vi "Control_laser_Main.vi"() -> ()   [LabVIEW 2024]
doc: "Use this template to build a simple state machine design pattern. Each state executes code and determines which state to transition to."
uses:
  controls/main_control State.ctl
  controls/main_control Data.ctl
  <vilib>/Utility/error.llb/DialogType.ctl
  <vilib>/DAQmx/create/channels.llb/DAQmx Create Channel (AI-Voltage-Basic).vi
  <vilib>/Utility/error.llb/Error Cluster From Error Code.vi
  <vilib>/ErrorRing/Error Ring.xnode
panel:
  in  "Laser diode control":bool
  out "Sweep Chart":dbl(graph)
  out "Laser Current (mA)":dbl
  out "Data Acq Iterations":i32
  in  "Connect DAQ":bool
  in  "Connect LD Control":bool
  out "Static acquisition Chart":dbl(graph)
  out "Standard deviation":dbl
  out "Mean":dbl
  in  "Mean iterations":i32
  in  "Stop Sweep":bool
  out "Sweep Running":bool
  out "Current Step":dbl format="%#_13g"
  in  "Final value (mA)":dbl format="%#_13g"
  in  "Interval (mA)":dbl format="%#_13g"
  in  "Initial value (mA)":dbl format="%#_13g"
  in  "Init Sweep":bool
  out "Steps":dbl format="%#_13g"
  in  "Data Acquisition":bool
  in  "Exit":bool
  in  "CH. AI Input":tag
  # "SWEEP PARAMETERS"
  # "STATIC ACQUISITION"
  # "LASER"
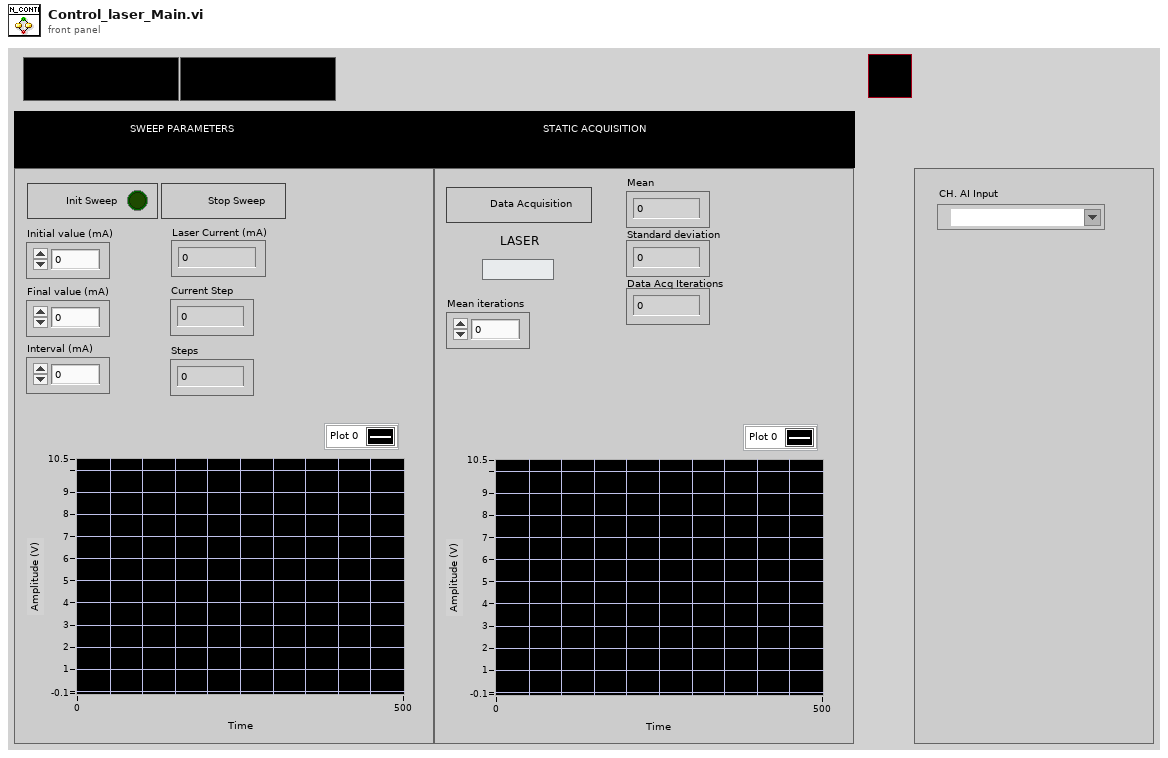
[diagram p1: front panel]
types:
  T1 = cluster{"Steps":refnum<vi>, "Current Step":refnum<vi>, "Final value (mA)":refnum<vi>, "Initial value (mA)":refnum<vi>, "Interval (mA)":refnum<vi>, "Data Acquisition":refnum<vi>, "Init Sweep":refnum<vi>, "Sweep Running":refnum<vi>, "Connect DAQ":refnum<vi>, "Connect LD Control":refnum<vi>}
  T2 = typedef "main_control Data.ctl" = cluster{"Boolean <Replace Me>":bool, "State":string, "Numeric <Replace Me>":dbl}
  T3 = typedef "main_control State.ctl" = enum16{"Initialize", "DAQ Handler", "LD Handler", "Wait for Event", "Data Acquisition", "Freq Sweep (Current)", "Error", "Exit"}
  T4 = typedef "DialogType.ctl" = u16
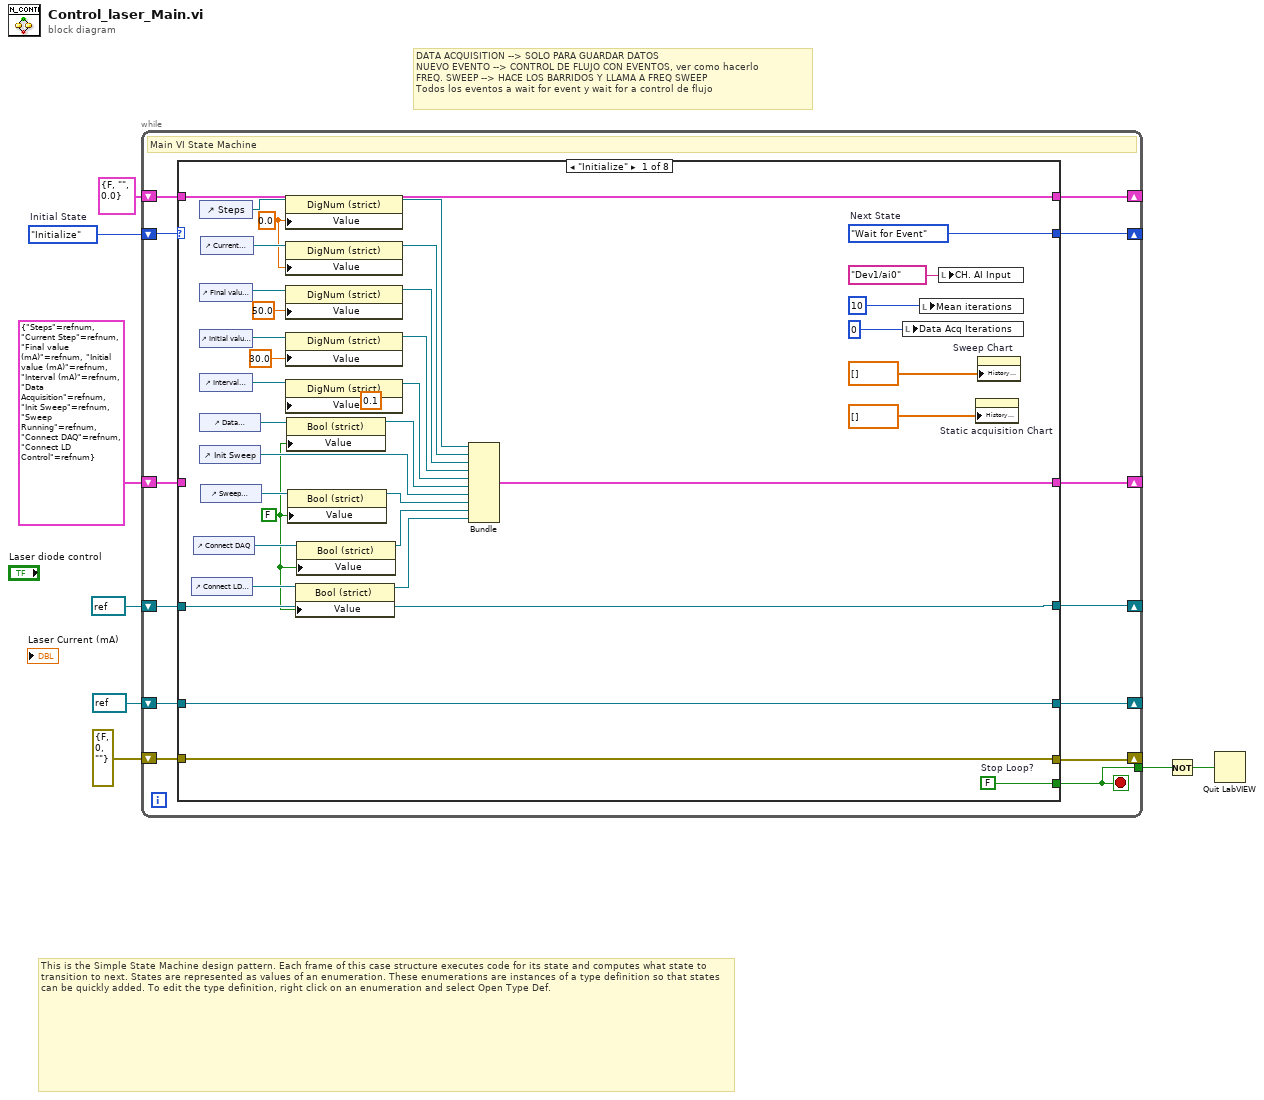
[diagram p0: block diagram]
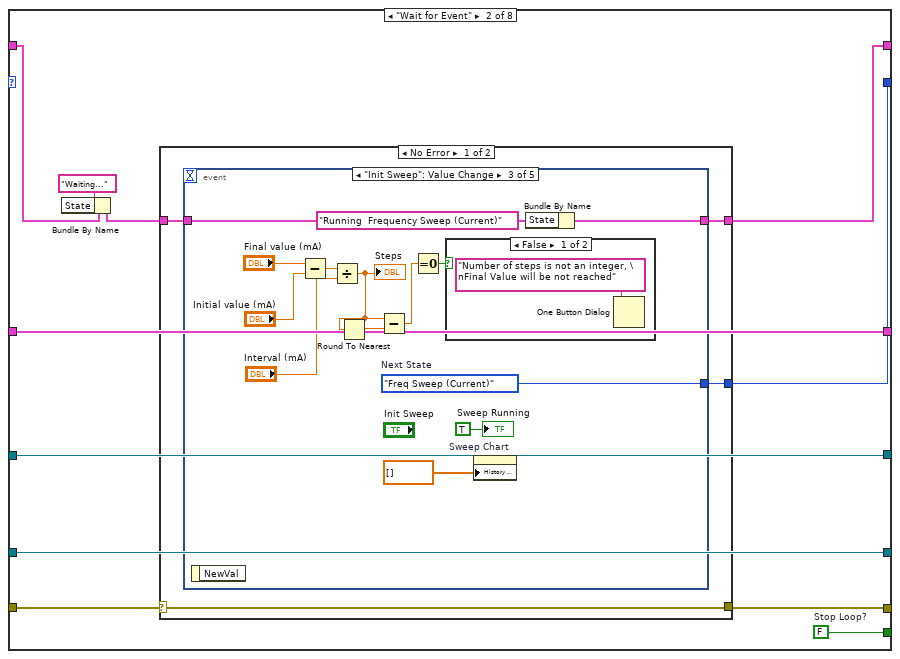
[diagram p2: hidden frame]
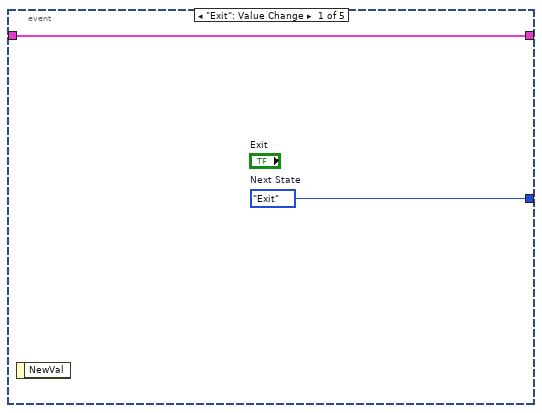
[diagram p3: hidden frame]
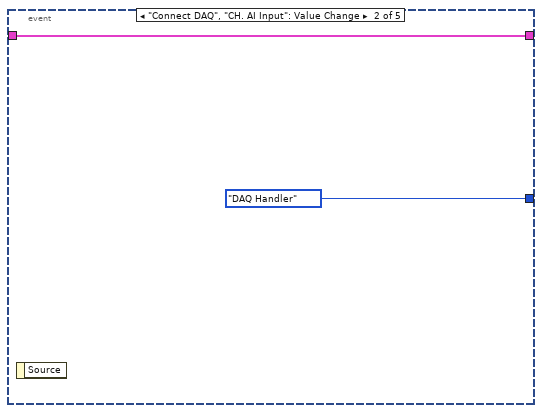
[diagram p4: hidden frame]
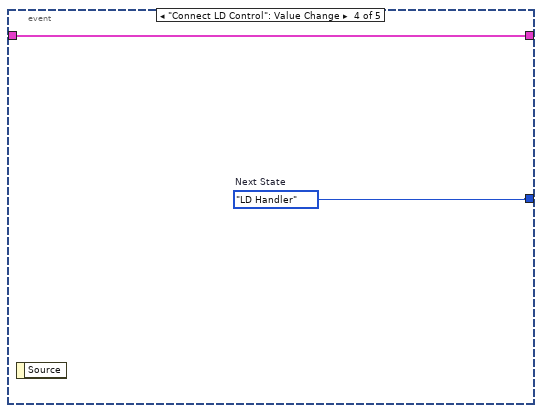
[diagram p6: hidden frame]
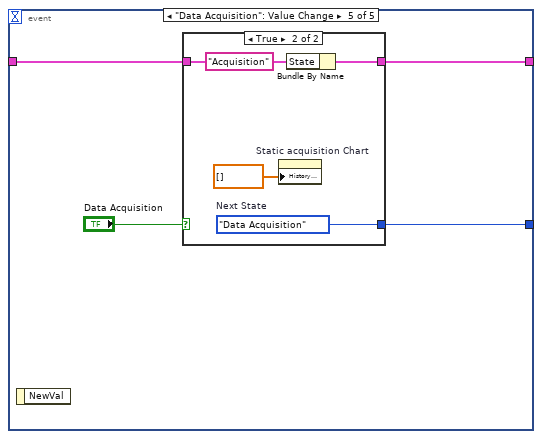
[diagram p7: hidden frame]
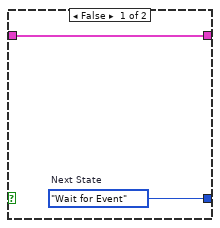
[diagram p8: hidden frame]
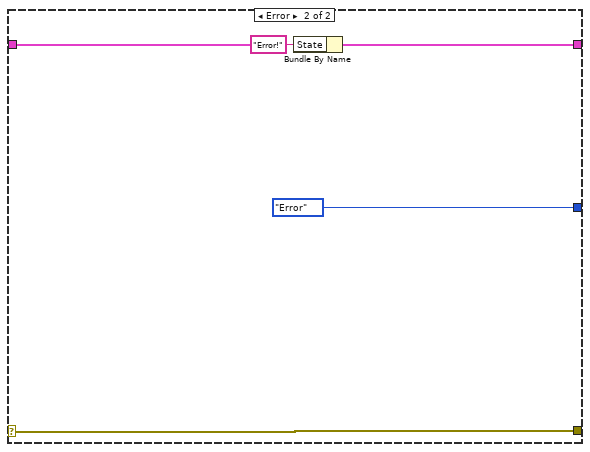
[diagram p9: hidden frame]
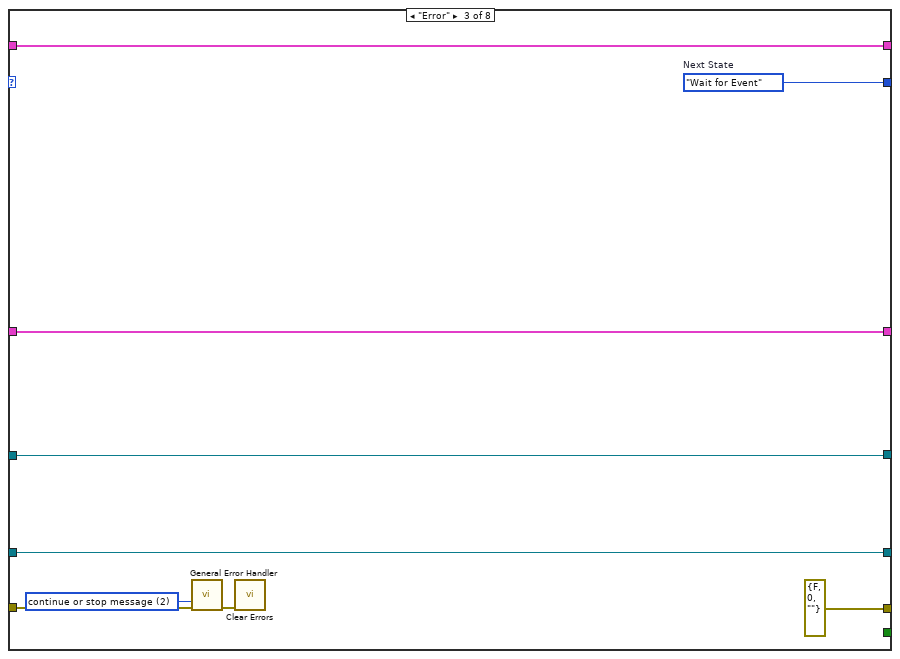
[diagram p10: hidden frame]
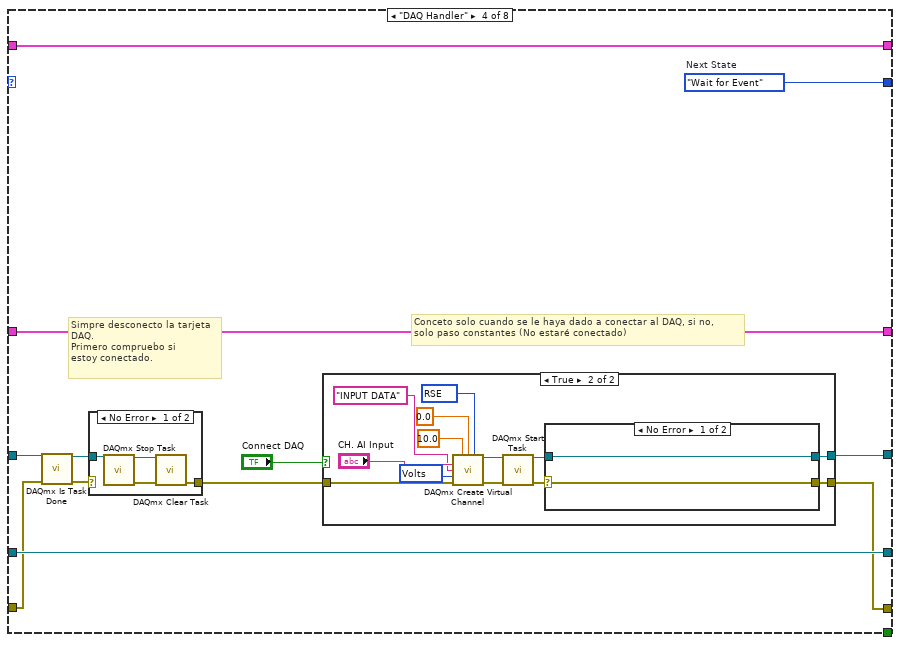
[diagram p11: hidden frame]
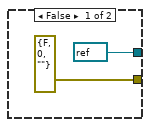
[diagram p12: hidden frame]
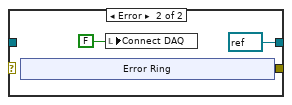
[diagram p13: hidden frame]
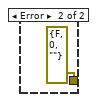
[diagram p14: hidden frame]
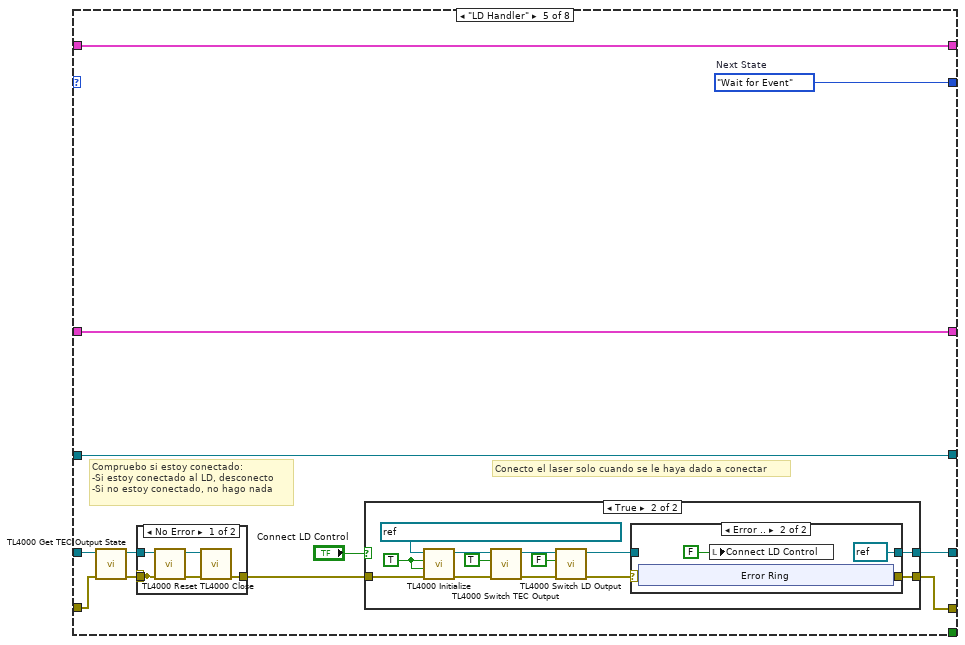
[diagram p15: hidden frame]
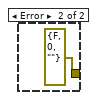
[diagram p16: hidden frame]
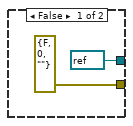
[diagram p17: hidden frame]
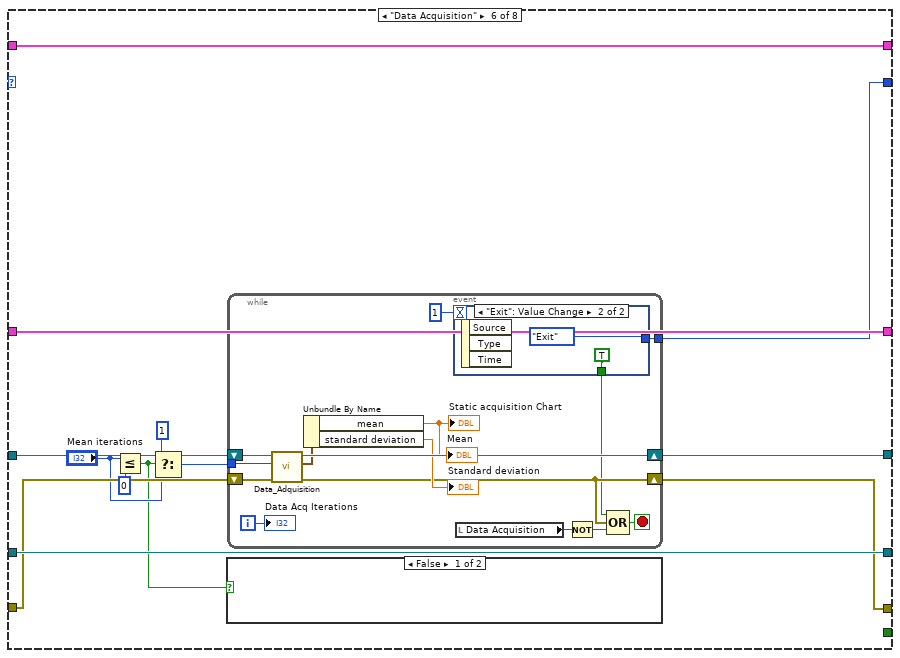
[diagram p19: hidden frame]
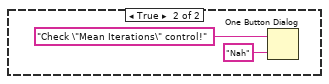
[diagram p20: hidden frame]
diagram:
  w8 = main_control_State."Initialize"  # Initial State
  # "DATA ACQUISITION --> SOLO PARA GUARDAR DATOS\nNUEVO EVENTO --> CONTROL DE FLUJO CON EVENTOS, ver como hacerlo\nFREQ. SWEEP --> HACE LOS BARRIDOS Y LLAMA A FREQ SWEEP\nTodos los eventos a wait for event y wait for a control de flujo"
  # "This is the Simple State Machine design pattern. Each frame of this case structure executes code for its state and computes what state to transition to next. States are represented as values of an enumeration. These enumerations are instances of a type definition so that states can be quickly added. To edit the type definition, right click on an enumeration and select Open Type Def."
  n1 = while {
    shift-right: [w20] -> _
    shift-left: w8 -> [w21]
    shift-right: [w18] -> _
    shift-left: T2 {"Boolean <Replace Me>"=FALSE, "State"="", "Numeric <Replace Me>"=0.0} ("Data") -> [w19]
    shift-right: [w17] -> _
    shift-left: refnum<visa-resource-name> refnum ("instrument handle out") -> [w14]
    shift-right: [w16] -> _
    shift-left: errorcluster {"status"=FALSE, "code"=0, "source"=""} ("error out") -> [w15]
    shift-right: [w12] -> _
    shift-left: T1 {"Steps"=refnum, "Current Step"=refnum, "Final value (mA)"=refnum, "Initial value (mA)"=refnum, "Interval (mA)"=refnum, "Data Acquisition"=refnum, "Init Sweep"=refnum, "Sweep Running"=refnum, "Connect DAQ"=refnum, "Connect LD Control"=refnum} -> [w13]
    shift-right: [w11] -> _
    shift-left: refnum<k21> refnum ("task out") -> [w10]
    tunnel: [w9] -> w3
    stop <- w9 stop-if-true
    # "Main VI State Machine"
    n2 = case shown="\"Initialize\"" w21 {
      tunnel: [w57 w68 w110 w127 w168 w211 w254 w316] -> w20
      tunnel: [w56 w67 _ _ _ _ _ w314] -> w9
      tunnel: w19 -> [w28 w59 w118 w130 w172 w216 w258 w315]
      tunnel: [w28 w66 w118 w130 w172 w216 w259 w315] -> w18
      tunnel: [w37 w65 w113 w128 w171 w214 w246 refnum<visa-resource-name> refnum ("VISA Refnum out")] -> w17
      tunnel: [w36 w61 errorcluster {"status"=FALSE, "code"=0, "source"=""} ("error IO") w120 w170 w209 w244 w312] -> w16
      tunnel: w15 -> [w36 w62 w117 w123 w166 w210 w252 w305]
      tunnel: w14 -> [w37 w65 w113 w128 w167 w214 w250 w308]
      tunnel: [w40 w63 w111 w121 w161 w215 w257 w313] -> w12
      tunnel: w13 -> [_ w63 w111 w121 w161 w215 w257 w313]
      tunnel: [w35 w64 w112 w129 w169 w213 w256 refnum<k21> refnum ("task out")] -> w11
      tunnel: w10 -> [w35 w64 w112 w125 w169 w212 w255 w303]
      frame "Initialize" {
        w24 = FALSE ("Value")
        w47 = 0.0
        w56 = FALSE  # Stop Loop?
        w57 = main_control_State."Wait for Event"  # Next State
        # "Initialize - Initialize the application."
        n3 = control-ref of="Connect LD Control"() -> (w25:refnum<vi>)
        n4 = control-ref of="Connect DAQ"() -> (w34:refnum<vi>)
        n5 = control-ref of="Steps"() -> (w55:refnum<vi>)
        n6 = control-ref of="Final value (mA)"() -> (w54:refnum<vi>)
        n7 = control-ref of="Initial value (mA)"() -> (w53:refnum<vi>)
        n8 = control-ref of="Interval (mA)"() -> (w52:refnum<vi>)
        n9 = control-ref of="Data Acquisition"() -> (w33:refnum<vi>)
        n10 = control-ref of="Init Sweep"() -> (w41:refnum<vi>)
        n11 = control-ref of="Current Step"() -> (w48:refnum<vi>)
        n12 = control-ref of="Sweep Running"() -> (w39:refnum<vi>)
        n13 = property class="DigNum (strict)"(reference=w55, "Value"=w47) -> (reference out=w46:refnum<vi>)  [unwired: 1 in, 1 out]
        n14 = property class="DigNum (strict)"(reference=w48, "Value"=w47) -> (reference out=w45:refnum<vi>)  [unwired: 1 in, 1 out]
        n15 = property class="DigNum (strict)"(reference=w54, "Value"=50.0) -> (reference out=w44:refnum<vi>)  [unwired: 1 in, 1 out]
        n16 = property class="DigNum (strict)"(reference=w53, "Value"=30.0) -> (reference out=w43:refnum<vi>)  [unwired: 1 in, 1 out]
        n17 = property class="DigNum (strict)"(reference=w52, "Value"=0.1) -> (reference out=w42:refnum<vi>)  [unwired: 1 in, 1 out]
        n18 = property class="Bool (strict)"(reference=w33, "Value"=w24) -> (reference out=w32:refnum<vi>)  [unwired: 1 in, 1 out]
        n19 = property class="Bool (strict)"(reference=w39, "Value"=w24) -> (reference out=w38:refnum<vi>)  [unwired: 1 in, 1 out]
        n20 = property class="Bool (strict)"(reference=w25, "Value"=w24) -> (reference out=w23:refnum<vi>)  [unwired: 1 in, 1 out]
        n21 = property class="Bool (strict)"(reference=w34, "Value"=w24) -> (reference out=w26:refnum<vi>)  [unwired: 1 in, 1 out]
        n22 = Bundle("Steps"=w46, "Current Step"=w45, "Final value (mA)"=w44, "Initial value (mA)"=w43, "Interval (mA)"=w42, "Data Acquisition"=w32, "Init Sweep"=w41, "Sweep Running"=w38, "Connect DAQ"=w26, "Connect LD Control"=w23) -> (w40:T1)  [unwired: 1 in]
        n23 = local write "Data Acq Iterations"(0 ("Data Acq Iterations")) -> ()
        n24 = local write "Mean iterations"(10 ("Mean iterations")) -> ()
        n25 = local write "CH. AI Input"(tag "Dev1/ai0" ("CH. AI Input")) -> ()
        n26 = property on="Static acquisition Chart" class="WFChart (strict)"("History Data"=dbl[] []) -> ()  [unwired: 2 in, 2 out]
        n27 = property on="Sweep Chart" class="WFChart (strict)"("History Data"=dbl[] []) -> ()  [unwired: 2 in, 2 out]
      }
      frame "Wait for Event" {
        w67 = FALSE  # Stop Loop?
        # "Wait for Event - Use an Event Structure to monitor the user interface for events that run different states of the state machine."
        n28 = Bundle By Name(cluster=w59, "State"="Waiting..." ("Running User State 1")) -> (w58:T2)
        n29 = case shown="No Error" w62 {
          selector: w62 -> [w70 w108]
          tunnel: [w72 main_control_State."Error" ("Next State")] -> w68
          tunnel: [w71 w105] -> w66
          tunnel: [w70 w108] -> w61
          tunnel: w58 -> [w69 w106]
          frame No Error {
            n30 = event shown="[2] \"Init Sweep\": Value Change" {
              selector: _ -> [_ _ _ _ _]
              dyn-events: _ -> [_ _ _ _ _]
              timeout: _ -> [_ _ _ _ _]
              tunnel: [w74 main_control_State."DAQ Handler" ("Next State") w90 w92 w97] -> w72
              tunnel: w69 -> [w73 w76 w89 w93 w96]
              tunnel: [w73 w76 w88 w93 w95] -> w71
              event "Exit": Value Change {
                w74 = main_control_State."Exit"  # Next State
                n31 = event-data() -> ()  [unwired: 1 in, 1 out]
              }
              event "Connect DAQ", "CH. AI Input": Value Change {
                n32 = event-data() -> ()  [unwired: 1 in, 1 out]
              }
              event "Init Sweep": Value Change {
                w90 = main_control_State."Freq Sweep (Current)"  # Next State
                n33 = event-data() -> ()  [unwired: 1 in, 1 out]
                n34 = Subtract(x="Final value (mA)", y="Initial value (mA)") -> (x-y=w85:dbl)
                n35 = Divide(x=w85, y="Interval (mA)") -> (x/y=w80:dbl)
                "Steps" <- w80
                n36 = Round To Nearest(number=w80) -> (nearest integer value=w81:dbl)
                n37 = Subtract(x=w80, y=w81) -> (x-y=w79:dbl)
                n38 = Equal To 0?(x=w79) -> (x = 0?=w78:bool)
                n39 = case shown="False" w78 {
                  frame False {
                    n40 = One Button Dialog(message="Number of steps is not an integer, \nFinal Value will be not reached") -> ()  [unwired: 1 in, 1 out]
                  }
                  frame True {
                  }
                }
                n41 = property on="Sweep Chart" class="WFChart (strict)"("History Data"=dbl[] []) -> ()  [unwired: 2 in, 2 out]
                n42 = Bundle By Name(cluster=w89, "State"="Running  Frequency Sweep (Current)" ("Running User State 1")) -> (w88:T2)
                "Sweep Running" <- TRUE ("Sweep Running")
              }
              event "Connect LD Control": Value Change {
                w92 = main_control_State."LD Handler"  # Next State
                n43 = event-data() -> ()  [unwired: 1 in, 1 out]
              }
              event "Data Acquisition": Value Change {
                n44 = event-data() -> ()  [unwired: 1 in, 1 out]
                n45 = case shown="True" "Data Acquisition" {
                  tunnel: [w99 w104] -> w97
                  tunnel: w96 -> [w98 w103]
                  tunnel: [w98 w101] -> w95
                  frame False {
                    w99 = main_control_State."Wait for Event"  # Next State
                  }
                  frame True {
                    w104 = main_control_State."Data Acquisition"  # Next State
                    n46 = property on="Static acquisition Chart" class="WFChart (strict)"("History Data"=dbl[] []) -> ()  [unwired: 2 in, 2 out]
                    n47 = Bundle By Name(cluster=w103, "State"="Acquisition" ("Running User State 2")) -> (w101:T2)
                  }
                }
              }
            }
          }
          frame Error {
            n48 = Bundle By Name(cluster=w106, "State"="Error!" ("Running User State 1")) -> (w105:T2)
          }
        }
      }
      frame "Error" {
        w110 = main_control_State."Wait for Event"  # Next State
        w116 = T4 2 items=["no dialog", "OK message", "continue or stop message", "OK message + warnings", "continue/stop + warnings"] ("type of dialog (OK msg:1)")
        n49 = call <vilib>:"General Error Handler.vi"("type of dialog (OK msg:1)"=w116, "error in (no error)"=w117) -> ("error out"=w115:errorcluster)  [unwired: 9 in, 4 out]
        n50 = call <vilib>:"Clear Errors.vi"("error in (no error)"=w115) -> ()  [unwired: 5 in, 2 out]
      }
      frame "DAQ Handler" {
        w127 = main_control_State."Wait for Event"  # Next State
        # "Simpre desconecto la tarjeta\nDAQ. \nPrimero compruebo si \nestoy conectado."
        # "Conceto solo cuando se le haya dado a conectar al DAQ, si no,\nsolo paso constantes (No estaré conectado)"
        n51 = call <vilib>:"DAQmx Is Task Done.vi"("task/channels in"=w125, "error in"=w123) -> ("task out"=w122:refnum<k21>, "error out"=w124:errorcluster)  [unwired: 11 in, 1 out]
        n52 = case shown="No Error" w124 {
          tunnel: [w157 errorcluster {"status"=FALSE, "code"=0, "source"=""} ("error out")] -> w126
          tunnel: w122 -> [w156 _]
          frame No Error {
            n53 = call <vilib>:"DAQmx Stop Task.vi"("task/channels in"=w156) -> ("task out"=w159:refnum<k21>, "error out"=w158:errorcluster)  [unwired: 13 in]
            n54 = call <vilib>:"DAQmx Clear Task.vi"("task in"=w159, "error in"=w158) -> ("error out"=w157:errorcluster)  [unwired: 13 in]
          }
          frame Error {
          }
        }
        n55 = case shown="True" "Connect DAQ" {
          tunnel: [refnum<k21> refnum ("task out") w134] -> w129
          tunnel: w126 -> [_ w137]
          tunnel: [errorcluster {"status"=FALSE, "code"=0, "source"=""} ("error out") w135] -> w120
          frame False {
          }
          frame True {
            w138 = 10348 items=["Volts"=10348, "From Custom Scale"=10065] ("units")
            w140 = 10083 items=["Default"=-1, "RSE"=10083, "NRSE"=10078, "Differential"=10106, "Pseudodifferential"=12529] ("input terminal configuration")
            n56 = call-poly <vilib>:"DAQmx Create Virtual Channel.vi"("maximum value"=10.0, "minimum value"=0.0, "input terminal configuration"=w140, "physical channels"="CH. AI Input", "name to assign"="INPUT DATA", "units"=w138, "error in"=w137) -> ("task out"=w143:refnum<k21>, "error out"=w144:errorcluster)  [unwired: 7 in]
            n57 = call <vilib>:"DAQmx Start Task.vi"("task/channels in"=w143, "error in"=w144) -> ("task out"=w133:refnum<k21>, "error out"=w136:errorcluster)  [unwired: 12 in]
            n58 = case shown="No Error" w136 {
              selector: w136 -> [w147 _]
              tunnel: [w147 w150] -> w135
              tunnel: [w146 refnum<k21> refnum ("task out")] -> w134
              tunnel: w133 -> [w146 _]
              frame No Error {
              }
              frame Error {
                n59 = xnode "Error Ring"() -> ("error out"=w150:errorcluster)
                n60 = local write "Connect DAQ"(FALSE ("Connect DAQ")) -> ()
              }
            }
          }
        }
      }
      frame "LD Handler" {
        w168 = main_control_State."Wait for Event"  # Next State
        # "Conecto el laser solo cuando se le haya dado a conectar"
        # "Compruebo si estoy conectado:\n-Si estoy conectado al LD, desconecto\n-Si no estoy conectado, no hago nada"
        n61 = call <instrlib>:"TL4000 Get TEC Output State.vi"("error in (no error)"=w166, "instrument handle"=w167) -> ("error out"=w164:errorcluster, "instrument handle out"=w165:refnum<visa-resource-name>)  [unwired: 7 in, 1 out]
        n62 = case shown="No Error" w164 {
          selector: w164 -> [w176 _]
          tunnel: w165 -> [w175 _]
          tunnel: w164 -> [_ _]
          tunnel: [w177 errorcluster {"status"=FALSE, "code"=0, "source"=""} ("error out")] -> w162
          frame No Error {
            n63 = call <instrlib>:"TL4000 Reset.vi"("error in (no error)"=w176, "instrument handle"=w175) -> ("error out"=w174:errorcluster, "instrument handle out"=w173:refnum<visa-resource-name>)  [unwired: 8 in]
            n64 = call <instrlib>:"TL4000 Close.vi"("error in (no error)"=w174, "instrument handle"=w173) -> ("error out"=w177:errorcluster)  [unwired: 9 in]
          }
          frame Error {
          }
        }
        n65 = case shown="True" "Connect LD Control" {
          tunnel: [refnum<visa-resource-name> refnum ("instrument handle out") w182] -> w171
          tunnel: [errorcluster {"status"=FALSE, "code"=0, "source"=""} ("error out") w183] -> w170
          tunnel: w162 -> [_ w185]
          frame False {
          }
          frame True {
            w187 = TRUE
            n66 = call <instrlib>:"TL4000 Initialize.vi"("error in (no error)"=w185, "Reset Device (Reset Device)"=w187, "ID Query (Do Query)"=w187, "resource name"=refnum<visa-resource-name> "USB0::0x1313::0x804F::M00287955::INSTR") -> ("error out"=w193:errorcluster, "instrument handle out"=w192:refnum<visa-resource-name>)  [unwired: 6 in]
            n67 = call <instrlib>:"TL4000 Switch TEC Output.vi"("error in (no error)"=w193, "TEC Output (Off)"=TRUE, "instrument handle"=w192) -> ("error out"=w190:errorcluster, "instrument handle out"=w191:refnum<visa-resource-name>)  [unwired: 7 in]
            n68 = call <instrlib>:"TL4000 Switch LD Output.vi"("error in (no error)"=w190, "LD Output (Off)"=FALSE, "instrument handle"=w191) -> ("error out"=w184:errorcluster, "instrument handle out"=w181:refnum<visa-resource-name>)  [unwired: 7 in]
            n69 = case shown="Error .." w184 {
              selector: w184 -> [w195 _]
              tunnel: [w195 w198] -> w183
              tunnel: [w194 refnum<visa-resource-name> refnum ("instrument handle out")] -> w182
              tunnel: w181 -> [w194 _]
              frame No Error {
              }
              frame Error {
                n70 = xnode "Error Ring"() -> ("error out"=w198:errorcluster)
                n71 = local write "Connect LD Control"(FALSE ("Connect LD Control")) -> ()
              }
            }
          }
        }
      }
      frame "Data Acquisition" {
        # "User State 1 - Replace this state with functionality for your own application."
        n72 = Less Or Equal?(x="Mean iterations", y=0) -> (x <= y?=w204:bool)
        n73 = Select(t=1, s=w204, f="Mean iterations") -> (s? t:f=w205:i32)
        n74 = case shown="False" w204 {
          frame False {
          }
          frame True {
            n75 = One Button Dialog(message="Check \"Mean Iterations\" control!", button name ("OK")="Nah") -> ()  [unwired: 1 out]
          }
        }
        n76 = while {
          shift-right: [w233] -> w213
          shift-left: w212 -> [w229]
          tunnel: [w221] -> w211
          shift-right: [w224] -> w209
          shift-left: w210 -> [w228]
          tunnel: w205 -> [w227]
          i -> [w230]
          stop <- w225 stop-if-true
          n77 = call "Data_Adquisition.vi"("error in"=w228, "Mean Iterations"=w227, "task in"=w229) -> ("error out"=w224:errorcluster, "mean and std"=w232:cluster{"mean":dbl, "standard deviation":dbl}, "task out"=w233:refnum<k21>)  [unwired: 3 in, 1 out]
          n78 = Unbundle By Name(w232) -> ("mean"=→"Mean" →"Static acquisition Chart":dbl, "standard deviation"=→"Standard deviation":dbl)
          n79 = event shown="[1] \"Exit\": Value Change" {
            selector: _ -> [_ _]
            dyn-events: _ -> [_ _]
            timeout: 1 -> [_ _]
            tunnel: [FALSE ("Data Acquisition") TRUE ("Data Acquisition")] -> w223
            tunnel: [main_control_State."Wait for Event" main_control_State."Exit"] -> w221
            event Timeout {
              n80 = event-data() -> ()  [unwired: 1 in, 3 out]
            }
            event "Exit": Value Change {
              n81 = event-data() -> ()  [unwired: 1 in, 3 out]
            }
          }
          n82 = local read "Data Acquisition"() -> (w220:bool)
          n83 = Not(x=w220) -> (.not. x?=w219:bool)
          n84 = Compound Arithmetic op=OR(w223, w224, w219) -> (w225:bool)
          "Data Acq Iterations" <- w230
        }
      }
      frame "Freq Sweep (Current)" {
        # "User State 2 - Replace this state with functionality for your own application."
        n85 = local read "Interval (mA)"() -> (w240:dbl)
        n86 = local read "Initial value (mA)"() -> (w242:dbl)
        n87 = local read "Steps"() -> (w239:dbl)
        n88 = call <instrlib>:"TL4000 Switch LD Output.vi"("error in (no error)"=w252, "LD Output (Off)"=TRUE, "instrument handle"=w250) -> ("error out"=w251:errorcluster, "instrument handle out"=w249:refnum<visa-resource-name>)  [unwired: 7 in]
        n89 = Divide(x=w242, y=1000.0) -> (x/y=w241:dbl)
        n90 = call "Reach_Current_Target.vi"("Amps"=w241) -> ()  [unwired: 8 in, 3 out]
        n91 = Bundle By Name(cluster=w258, "State"="Acquisition" ("Running User State 2")) -> (w259:T2)
        n92 = while {
          shift-right: [w273] -> w245
          shift-left: w251 -> [w283]
          tunnel: [w275] -> w254
          shift-right: [w277] -> w256
          shift-left: w255 -> [w276]
          shift-right: [w279] -> w247
          shift-left: w249 -> [w284]
          tunnel: w242 -> [w266]
          tunnel: w240 -> [w265]
          tunnel: w239 -> [w264]
          tunnel: [0.0 ("Current Step")] -> w238
          stop <- w271 stop-if-true
          # "Aumento la corriente según\nel intervalo establecido"
          n93 = local read "Current Step"() -> (w263:dbl)
          n94 = Increment(x=w263) -> (x+1=w262:dbl)
          n95 = Multiply(x=w263, y=w265) -> (x*y=w282:dbl)
          n96 = Greater?(x=w262, y=w264) -> (0:w269:bool)
          n97 = Add(x=w282, y=w266) -> (x+y=w280:dbl)
          n98 = Divide(x=w280, y=1000.0) -> (x/y=w278:dbl)
          n99 = call "Reach_Current_Target.vi"("error in (no error)"=w283, "Amps"=w278, "VISA Refnum in"=w284) -> ("error out"=w274:errorcluster, "Laser current"=w267:dbl, "VISA Refnum out"=w279:refnum<visa-resource-name>)  [unwired: 6 in]
          n100 = local write "Laser Current (mA)"(w267) -> ()
          n101 = case shown="No Error" w274 {
            selector: w274 -> [_ w293]
            tunnel: [w292 w294] -> w277
            tunnel: w276 -> [w291 w294]
            tunnel: [w288 w293] -> w273
            tunnel: w263 -> [w286 _]
            frame No Error {
              n102 = Increment(x=w286) -> (x+1=→"Current Step":dbl)
              n103 = local read "Mean iterations"() -> (w290:i32)
              n104 = call "Data_Adquisition.vi"("Mean Iterations"=w290, "task in"=w291) -> ("error out"=w288:errorcluster, "mean and std"=w289:cluster{"mean":dbl, "standard deviation":dbl}, "task out"=w292:refnum<k21>)  [unwired: 4 in, 1 out]
              n105 = Unbundle By Name(w289) -> ("mean"=→"Sweep Chart":dbl)
            }
            frame Error {
            }
          }
          n106 = event shown="[0] \"Stop Sweep\": Value Change" {
            selector: _ -> [_ _ _]
            dyn-events: _ -> [_ _ _]
            timeout: 100 -> [_ _ _]
            tunnel: [TRUE ("s") FALSE ("s") TRUE ("s")] -> w272
            tunnel: [main_control_State."Wait for Event" ("Next State") main_control_State."Wait for Event" ("Next State") main_control_State."Exit" ("Next State")] -> w275
            event "Stop Sweep": Value Change {
              n107 = event-data() -> ()  [unwired: 1 in, 2 out]
            }
            event Timeout {
              n108 = event-data() -> ()  [unwired: 1 in, 3 out]
            }
            event "Exit": Value Change {
              n109 = event-data() -> ()  [unwired: 1 in, 2 out]
            }
          }
          n110 = Compound Arithmetic op=OR(w273, w272, w269) -> (w271:bool)
          n111 = Not(x=w271) -> (.not. x?=w270:bool)
          n112 = local write "Sweep Running"(w270) -> ()
        }
        n113 = local write "Current Step"(w238) -> ()
        n114 = call <instrlib>:"TL4000 Switch LD Output.vi"("error in (no error)"=w245, "LD Output (Off)"=FALSE, "instrument handle"=w247) -> ("error out"=w244:errorcluster, "instrument handle out"=w246:refnum<visa-resource-name>)  [unwired: 7 in]
      }
      frame "Exit" {
        w314 = TRUE  # Stop Loop?
        w316 = main_control_State."Exit"  # (Value Not Used)
        # "The state value is not used here since this is the last iteration of the state machine loop."
        # "Exit - Exit the application."
        n115 = call <instrlib>:"TL4000 Measure Temperature.vi"("instrument handle"=w308) -> ("error out"=w306:errorcluster, "instrument handle out"=w307:refnum<visa-resource-name>)  [unwired: 8 in, 1 out]
        n116 = case shown="No Error" w306 {
          selector: w306 -> [w317 _]
          tunnel: w307 -> [w318 _]
          tunnel: [w317 errorcluster {"status"=FALSE, "code"=0, "source"=""} ("error out")] -> w304
          frame No Error {
            n117 = call <instrlib>:"TL4000 Switch TEC Output.vi"("TEC Output (Off)"=FALSE, "instrument handle"=w318) -> ("instrument handle out"=w322:refnum<visa-resource-name>)  [unwired: 8 in, 1 out]
            n118 = call <instrlib>:"TL4000 Switch LD Output.vi"("LD Output (Off)"=FALSE, "instrument handle"=w322) -> ("instrument handle out"=w319:refnum<visa-resource-name>)  [unwired: 8 in, 1 out]
            n119 = call <instrlib>:"TL4000 Reset.vi"("instrument handle"=w319) -> ("instrument handle out"=w323:refnum<visa-resource-name>)  [unwired: 9 in, 1 out]
            n120 = call <instrlib>:"TL4000 Close.vi"("instrument handle"=w323) -> ()  [unwired: 10 in, 1 out]
          }
          frame Error {
          }
        }
        n121 = call <vilib>:"DAQmx Is Task Done.vi"("task/channels in"=w303) -> ("task out"=w302:refnum<k21>, "error out"=w301:errorcluster)  [unwired: 12 in, 1 out]
        n122 = case shown="Error .." w301 {
          tunnel: [w326 errorcluster {"status"=FALSE, "code"=0, "source"=""} ("error out")] -> w309
          tunnel: w302 -> [w325 _]
          frame No Error {
            n123 = call <vilib>:"DAQmx Stop Task.vi"("task/channels in"=w325) -> ("task out"=w328:refnum<k21>, "error out"=w327:errorcluster)  [unwired: 13 in]
            n124 = call <vilib>:"DAQmx Clear Task.vi"("task in"=w328, "error in"=w327) -> ("error out"=w326:errorcluster)  [unwired: 13 in]
          }
          frame Error {
          }
        }
        n125 = Merge Errors(w309, w304, w305) -> (w312:errorcluster)
      }
    }
  }
  n126 = Not(x=w3) -> (.not. x?=w2:bool)
  n127 = Quit LabVIEW(quit? (T)=w2) -> ()
